vi "Message References to Message Handles.vi"(8 "error in":errorcluster, 11 "message refs":T3[](array[typedef]) format="%.0x") -> (0 "error out":errorcluster, 3 "message handles":T1 {"Rx status handles" format="%.0x"; "Tx status handles" format="%.0x"; "timestamps" format="%.0x"; "parameters"."RxBC channel handle" format="%.0x"; "parameters"."RxRT channel handle" format="%.0x"; "parameters"."Tx channel handle" format="%.0x"})   [LabVIEW 2020, in "AIM MIL-STD-1553 Engine.lvlib" / "Implementation.lvlib" / "Execution Unit.lvclass"]
uses:
  Execution Unit.lvclass
  <vilib>/NI VeriStand/Custom Device API/Custom Device Item Ref.ctl
  Message Handles.ctl
  Parameter Handles.ctl
  <vilib>/NI VeriStand/Custom Device API/Custom Device API.lvlib
  Scripting/AIM MIL-STD-1553 Scripting.lvlib
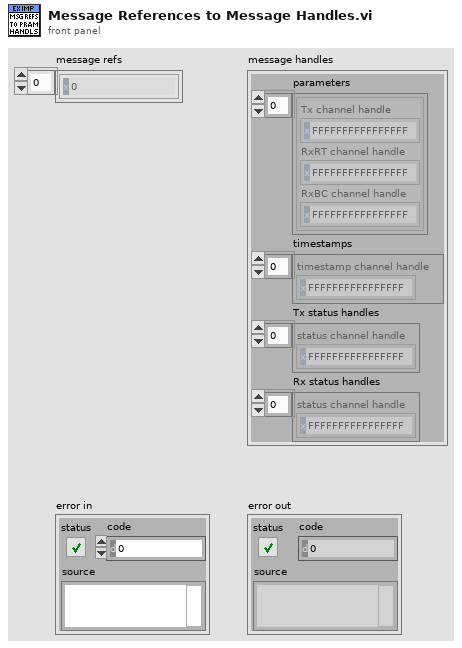
[diagram p1: front panel]
types:
  T1 = typedef "AIM MIL-STD-1553 Engine.lvlib/Implementation.lvlib/Execution Unit.lvclass/Message Handles.ctl" = cluster{"parameters":T2[], "timestamps":T3[], "Tx status handles":T3[], "Rx status handles":T3[]}
  T2 = typedef "AIM MIL-STD-1553 Engine.lvlib/Implementation.lvlib/Execution Unit.lvclass/Parameter Handles.ctl" = cluster{"Tx channel handle":T3, "RxRT channel handle":T3, "RxBC channel handle":T3}
  T3 = typedef "Custom Device API.lvlib/Custom Device Item Ref.ctl" = u64
  T4 = typedef "Direction.ctl" = enum16{"Rx", "Tx"}
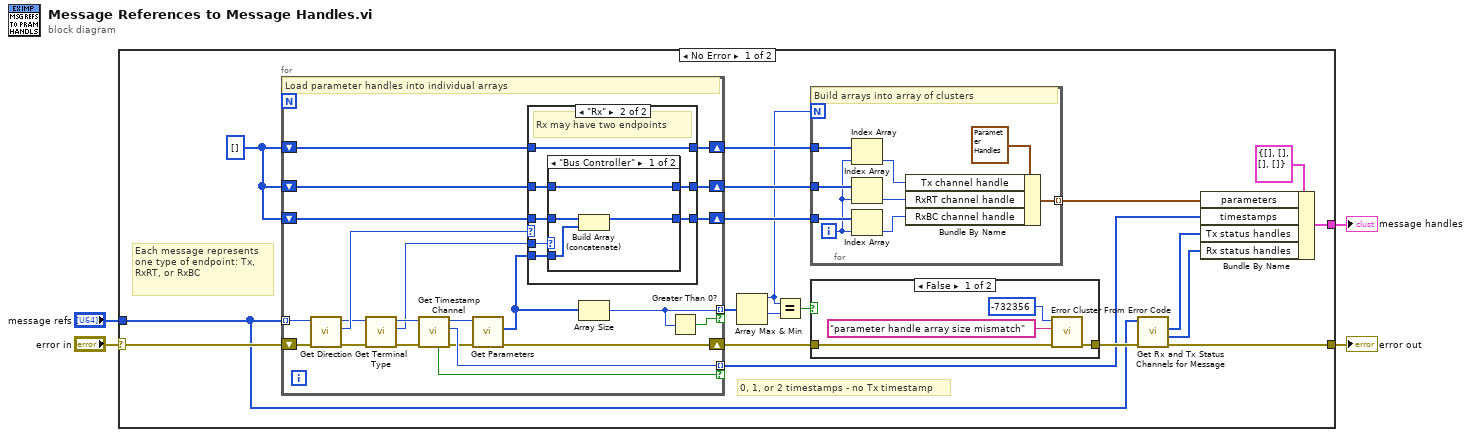
[diagram p0: block diagram]
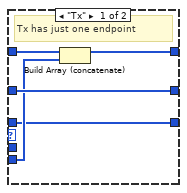
[diagram p2: hidden frame]
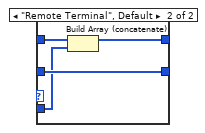
[diagram p3: hidden frame]
diagram:
  n1 = case shown="No Error" "error in" {
    selector: "error in" -> [w20 w80]
    tunnel: [w15 w80] -> w3
    tunnel: "message refs" -> [w12 _]
    tunnel: [w19 _] -> w1
    frame No Error {
      w17 = T3[] [] ("parameters")
      # "0, 1, or 2 timestamps - no Tx timestamp"
      # "Each message represents one type of endpoint: Tx, RxRT, or RxBC"
      n2 = for {
        shift-right: [w26] -> w21
        shift-left: w20 -> [w39]
        tunnel: w12 -> [w38] mode=indexing
        shift-right: [w40] -> w8
        shift-left: w17 -> [w45]
        shift-right: [w41] -> w9
        shift-left: w17 -> [w44]
        shift-right: [w42] -> w10
        shift-left: w17 -> [w43]
        tunnel: [w33] -> w22 mode=indexing if=w34
        tunnel: [w32] -> w11 mode=indexing if=w31
        # "Load parameter handles into individual arrays"
        n3 = call "Get Direction.vi"("error in"=w39, "message in"=w38) -> ("error out"=w35:errorcluster, "direction"=w37:T4, "message out"=w36:T3)  [unwired: 6 in, 1 out]
        n4 = call "Get Terminal Type.vi"("error in"=w35, "message in"=w36) -> ("error out"=w29:errorcluster, "terminal type"=w24:enum16{"Bus Controller", "Remote Terminal"}, "message out"=w30:T3)  [unwired: 7 in]
        n5 = call "Get Timestamp Channel.vi"("error in"=w29, "message in"=w30) -> ("error out"=w27:errorcluster, "timestamp channel"=w32:T3, "message out"=w28:T3, "found?"=w31:bool)  [unwired: 6 in]
        n6 = call "Get Parameters.vi"("error in"=w27, "message in"=w28) -> ("error out"=w26:errorcluster, "parameters"=w25:T3[])  [unwired: 7 in, 1 out]
        n7 = case shown="\"Rx\"" w37 {
          tunnel: w25 -> [w47 w51]
          tunnel: w45 -> [w46 w55]
          tunnel: w44 -> [w50 w53]
          tunnel: w43 -> [w49 w56]
          tunnel: [w48 w56] -> w42
          tunnel: [w50 w52] -> w41
          tunnel: [w46 w54] -> w40
          tunnel: w24 -> [_ w57]
          frame "Tx" {
            # "Tx has just one endpoint"
            n8 = Build Array (concatenate)(w49, w47) -> (w48:T3[])
          }
          frame "Rx" {
            # "Rx may have two endpoints"
            n9 = case shown="\"Bus Controller\"" w57 {
              tunnel: w55 -> [w61 w65]
              tunnel: [w60 w65] -> w54
              tunnel: w53 -> [w58 w64]
              tunnel: [w58 w63] -> w52
              tunnel: w51 -> [w59 w62]
              frame "Bus Controller" {
                # "TA is 0 for BC"
                n10 = Build Array (concatenate)(w61, w59) -> (w60:T3[])
              }
              frame "Remote Terminal", Default {
                # "TA is nonzero for RT"
                n11 = Build Array (concatenate)(w64, w62) -> (w63:T3[])
              }
            }
          }
        }
        n12 = Array Size(array=w25) -> (size(s)=w33:i32)
        n13 = Greater Than 0?(x=w33) -> (x > 0?=w34:bool)
      }
      n14 = Array Max & Min(array=w22) -> (max value=w5:i32, min value=w7:i32)  [unwired: 2 out]
      n15 = Equal?(x=w5, y=w7) -> (x = y?=w6:bool)
      n16 = for {
        N: w5 -> [_]
        tunnel: w10 -> [w79]
        tunnel: w9 -> [w78]
        tunnel: w8 -> [w77]
        tunnel: [w73] -> w23 mode=indexing
        i -> [w72]
        # "Build arrays into array of clusters"
        n17 = Index Array(array=w79, index=w72) -> (element=w76:T3)
        n18 = Index Array(array=w78, index=w72) -> (element=w75:T3)
        n19 = Index Array(array=w77, index=w72) -> (element=w74:T3)
        n20 = Bundle By Name(cluster=T2 {"Tx channel handle"=18446744073709551615, "RxRT channel handle"=18446744073709551615, "RxBC channel handle"=18446744073709551615} ("parameter handles"), "Tx channel handle"=w76, "RxRT channel handle"=w75, "RxBC channel handle"=w74) -> (w73:T2)
      }
      n21 = case shown="False" w6 {
        tunnel: [w69 w70] -> w16
        tunnel: w21 -> [w67 w70]
        frame False {
          n22 = call <vilib>:"Error Cluster From Error Code.vi"("error in (no error)"=w67, "error message (\"\")"="parameter handle array size mismatch" ("format string"), "error code (0)"=-732356) -> ("error out"=w69:errorcluster)  [unwired: 6 in]
        }
        frame True {
        }
      }
      n23 = call "Get Rx and Tx Status Channels for Message.vi"("error in"=w16, "message refs"=w12) -> ("error out"=w15:errorcluster, "Rx status channels"=w13:T3[], "Tx status channels"=w14:T3[])  [unwired: 6 in, 1 out]
      n24 = Bundle By Name(cluster=T1 {"parameters"=[], "timestamps"=[], "Tx status handles"=[], "Rx status handles"=[]} ("message handles"), "parameters"=w23, "timestamps"=w11, "Tx status handles"=w14, "Rx status handles"=w13) -> (w19:T1)
    }
    frame Error {
    }
  }
  "error out" <- w3
  "message handles" <- w1
